vi "Previous Button Init.vi"(3 "Container State":T3, 4 "Previous State":variant, 5 "Previous Version":T2) -> (2 "Current State":T1)   [LabVIEW 2009, in "Previous Button (Modern).xctl"]
uses:
  <vilib>/Navigation Controls/Previous Button/Previous Button (Modern).xctl
  <vilib>/Navigation Controls/Previous Button/Previous Button State.ctl
  <vilib>/_xctls/Container State.ctl
  <vilib>/_xctls/Version.ctl
  <vilib>/Navigation Controls/NI_Navigation.lvlib
  <vilib>/_xctls/XControlSupport.lvlib
panel:
  in  "Default Indicator State":T1
  in  "Default Control State":T1
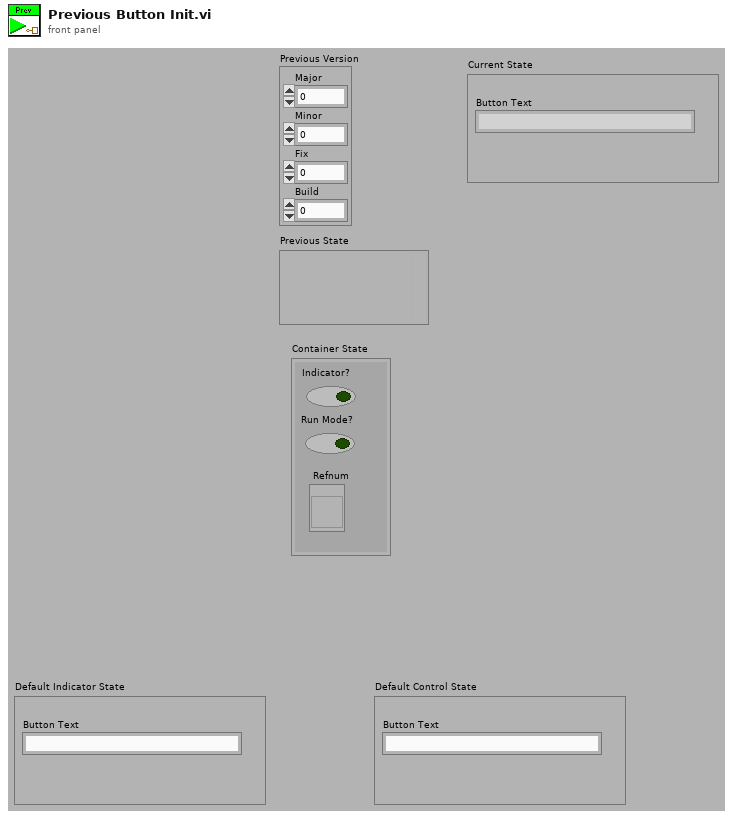
[diagram p1: front panel]
types:
  T1 = typedef "Previous Button (Modern).xctl/Previous Button State.ctl" = cluster{"Button Text":string}
  T2 = typedef "XControlSupport.lvlib/Version.ctl" = cluster{"Major":u16, "Minor":u16, "Fix":u16, "Build":u16}
  T3 = typedef "XControlSupport.lvlib/Container State.ctl" = cluster{"Indicator?":bool, "Run Mode?":bool, " Refnum":refnum<vi>}
  T4 = enum32{"Next Modern", "Next System", "Previous Modern", "Previous System", "Jump Modern", "Jump System", "N/A"}
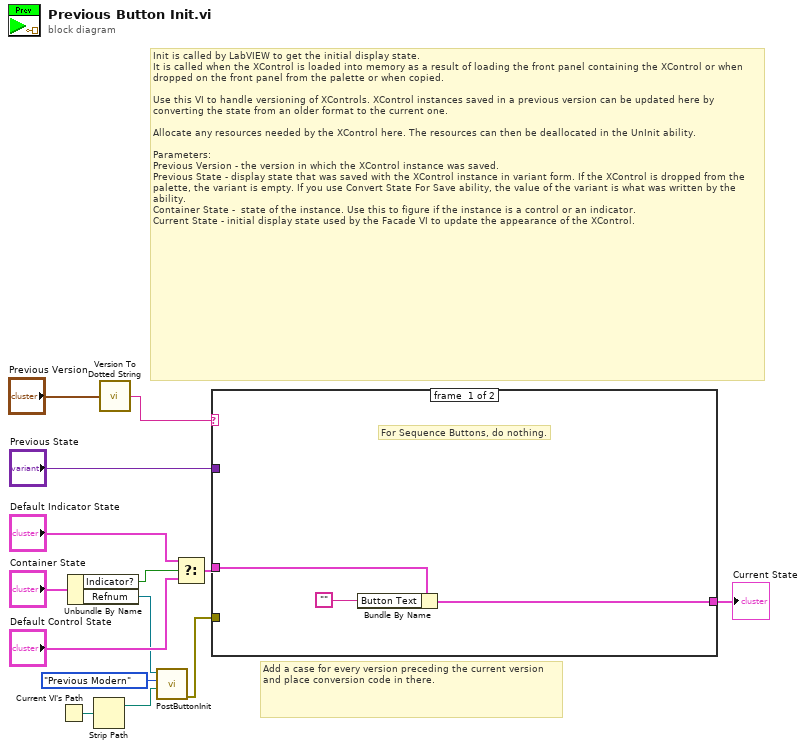
[diagram p0: block diagram]
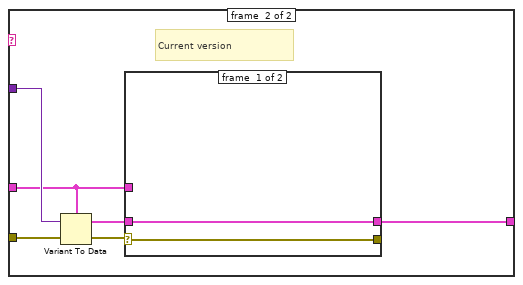
[diagram p2: hidden frame]
diagram:
  # "Add a case for every version preceding the current version and place conversion code in there."
  # "Init is called by LabVIEW to get the initial display state.\nIt is called when the XControl is loaded into memory as a result of loading the front panel containing the XControl or when dropped on the front panel from the palette or when copied.\n\nUse this VI to handle versioning of XControls. XControl instances saved in a previous version can be updated here by converting the state from an older format to the current one.\n\nAllocate any resources needed by the XControl here. The resources can then be deallocated in the UnInit ability.\n\nParameters:\nPrevious Version - the version in which the XControl instance was saved.\nPrevious State - display state that was saved with the XControl instance in variant form. If the XControl is dropped from the palette, the variant is empty. If you use Convert State For Save ability, the value of the variant is what was written by the ability. \nContainer State -  state of the instance. Use this to figure if the instance is a control or an indicator.\nCurrent State - initial display state used by the Facade VI to update the appearance of the XControl."
  n1 = Current VI's Path() -> (path=w2:path)
  n2 = Unbundle By Name("Container State") -> ("Indicator?"=w9:bool, "Refnum"=w5:refnum<vi>)
  n3 = Strip Path(path=w2) -> (stripped path=w1:path)  [unwired: 1 out]
  n4 = call <vilib>:"Version To Dotted String.vi"("Version"="Previous Version") -> ("String Version"=w6:string)
  n5 = call <vilib>:"PostButtonInit.vi"("Current Path"=w1, "Button Type"=T4."Previous Modern", "Control Refnum"=w5) -> ("error out"=w3:errorcluster)  [unwired: 7 in, 1 out]
  n6 = Select(t="Default Indicator State", s=w9, f="Default Control State") -> (s? t:f=w8:T1)
  n7 = case shown="\"1.0.0.0\"" w6 {
    tunnel: "Previous State" -> [_ w23]
    tunnel: [w15 w19] -> w13
    tunnel: w8 -> [w17 w20]
    tunnel: w3 -> [_ w18]
    frame #0 {
      # "For Sequence Buttons, do nothing."
      n8 = Bundle By Name(cluster=w17, "Button Text"="") -> (w15:T1)
    }
    frame #1 {
      # "Current version"
      n9 = Variant To Data(error in=w18, Variant=w23, type=w20) -> (error out=w22:errorcluster, data=w21:T1)
      n10 = case shown="No Error" w22 {
        selector: w22 -> [w25 w26]
        tunnel: w21 -> [w24 _]
        tunnel: [w24 w27] -> w19
        tunnel: w20 -> [_ w27]
        tunnel: [w25 w26] -> _
        frame #0 {
        }
        frame #1 {
          # "Error converting previously \nsaved state. Use default instead."
        }
      }
    }
  }
  "Current State" <- w13
